vi "Wait Function.vi"(8 "error in (no error)":errorcluster, 11 "Wait (ms)":u32) -> (0 "error out":errorcluster)   [LabVIEW 2024, in "Shared Steps.lvlib"]
uses:
  Shared Steps.lvlib
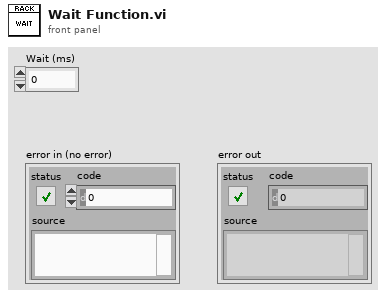
[diagram p1: front panel]
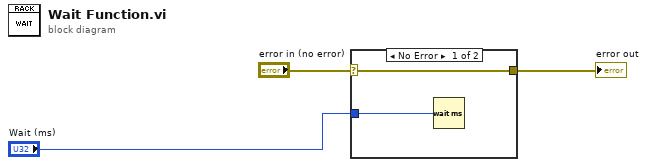
[diagram p0: block diagram]
diagram:
  n1 = case shown="No Error" "error in (no error)" {
    selector: "error in (no error)" -> [w5 w6]
    tunnel: [w5 w6] -> w2
    tunnel: "Wait (ms)" -> [w4 _]
    frame No Error {
      n2 = Wait (ms)(milliseconds to wait=w4) -> ()  [unwired: 1 out]
    }
    frame Error {
    }
  }
  "error out" <- w2
